vi "Open File Explorer.vi"(8 "error in (no error)":errorcluster, 11 "Full Path":path) -> (0 "error out":errorcluster)   [LabVIEW 2020, in "RxnRover.lvlib" / "File IO.lvlib"]
doc: "Opens up the file explorer to a location given in a file path (absolute)\nDoes this by sending a command into the command terminal, supports Windows, Mac OS, and Linux\n\nCreated 5/30/2025\nRxnRover"
uses:
  File IO.lvlib
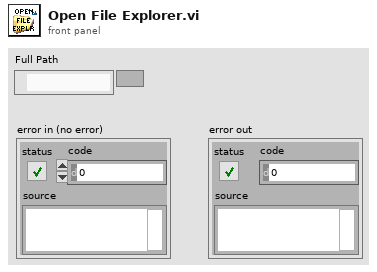
[diagram p1: front panel]
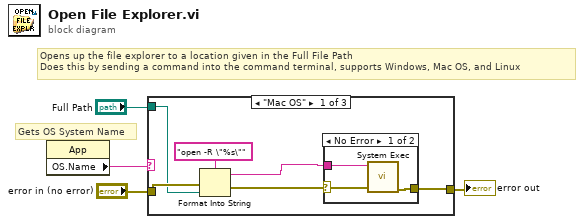
[diagram p0: block diagram]
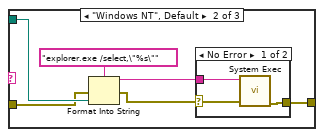
[diagram p3: hidden frame]
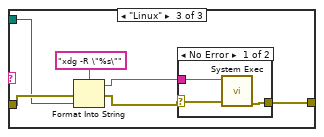
[diagram p5: hidden frame]
diagram:
  # "Opens up the file explorer to a location given in the Full File Path\nDoes this by sending a command into the command terminal, supports Windows, Mac OS, and Linux"
  # "Gets OS System Name"
  n1 = property class="App"() -> ("OS.Name"=w2:string)  [unwired: 2 in, 2 out]
  n2 = case shown="\"Mac OS\"" w2 {
    tunnel: "error in (no error)" -> [w10 w17 w30]
    tunnel: [w5 w15 w25] -> w4
    tunnel: "Full Path" -> [w9 w19 w29]
    frame "Mac OS" {
      n3 = Format Into String(format string="open -R \"%s\"", error in=w10, w9) -> (resulting string=w7:string, error out=w6:errorcluster)  [unwired: 1 in]
      n4 = case shown="No Error" w6 {
        selector: w6 -> [w12 w14]
        tunnel: [w11 w14] -> w5
        tunnel: w7 -> [w13 _]
        frame No Error {
          n5 = call <vilib>:"System Exec.vi"("error in (no error)"=w12, "command line"=w13) -> ("error out"=w11:errorcluster)  [unwired: 6 in, 3 out]
        }
        frame Error {
        }
      }
    }
    frame "Windows NT", Default {
      n6 = Format Into String(format string="explorer.exe /select,\"%s\"", error in=w17, w19) -> (resulting string=w20:string, error out=w16:errorcluster)  [unwired: 1 in]
      n7 = case shown="No Error" w16 {
        selector: w16 -> [w22 w24]
        tunnel: [w21 w24] -> w15
        tunnel: w20 -> [w23 _]
        frame No Error {
          n8 = call <vilib>:"System Exec.vi"("error in (no error)"=w22, "command line"=w23) -> ("error out"=w21:errorcluster)  [unwired: 6 in, 3 out]
        }
        frame Error {
        }
      }
    }
    frame "Linux" {
      n9 = Format Into String(format string="xdg -R \"%s\"", error in=w30, w29) -> (resulting string=w27:string, error out=w26:errorcluster)  [unwired: 1 in]
      n10 = case shown="No Error" w26 {
        selector: w26 -> [w32 w34]
        tunnel: [w31 w34] -> w25
        tunnel: w27 -> [w33 _]
        frame No Error {
          n11 = call <vilib>:"System Exec.vi"("error in (no error)"=w32, "command line"=w33) -> ("error out"=w31:errorcluster)  [unwired: 6 in, 3 out]
        }
        frame Error {
        }
      }
    }
  }
  "error out" <- w4
